vi "test Loopback with Disable.vi"(8 "error in":errorcluster, 11 "TestCase in":refnum<class "SingleCore.lvclass">) -> (0 "error out":errorcluster, 3 "TestCase out":refnum<class "SingleCore.lvclass">)   [LabVIEW 2020, in "SingleCore.lvclass"]
uses:
  SingleCore.lvclass
  C:/Git/niveristand-custom-device-testing-tools/VeriStandTestCase/VeriStandTestCase.lvclass
  4b06c685-66bb-4135-9ad1-d89a50a95502.vi
  <vilib>/numeric/Random Number (Range) I64.vi
  4cc353ea-8eb2-4b69-8f0e-bf7f0ec9a5d6.vi
  2771a990-9a12-45e1-bfa9-cf8078c77ee0.vi
  97c2081a-a4c0-4f2f-8a1c-7834fbf3da42.vi
  194ce8b8-c6d7-4123-a4fb-3c321acd640d.vi
  f114cf08-2618-4622-be37-923f8c3475b2.vi
  639b215b-9681-4d6c-ae13-b880b31cf4b5.vi
  f8fda0d9-e382-4aa3-871a-597408bfcf2f.vi
  <vilib>/numeric/sub_Random U32.vi
  <vilib>/NI VeriStand/Execution/Workspace/NI VeriStand - Set Multiple Channel Values.vi
  <vilib>/NI VeriStand/Execution/Workspace/NI VeriStand - Get Multiple Channel Values.vi
  <vilib>/addons/_JKI Toolkits/VI Tester/TestCase.llb/TestCase.lvclass
  <vilib>/NI VeriStand/Execution/Workspace/NI_VS Workspace ExecutionAPI.lvlib
  C:/Program Files (x86)/National Instruments/LabVIEW 2020/vi.lib/addons/_JKI Toolkits/VI Tester/TestCase.llb/TestCase.lvclass
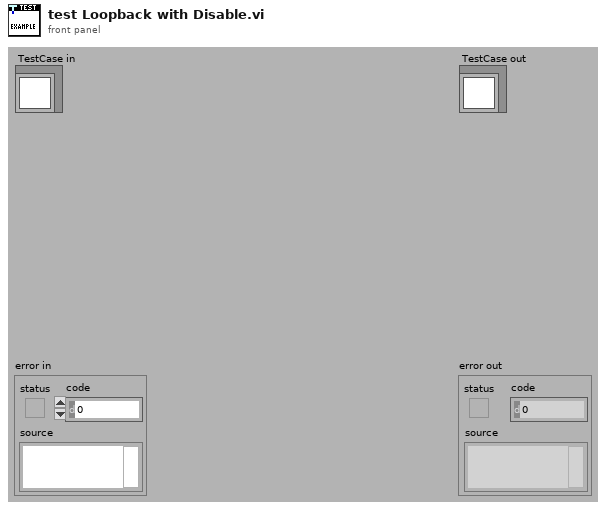
[diagram p1: front panel]
types:
  T1 = typedef "NI_VS Workspace ExecutionAPI.lvlib/WorkspaceAPI.ctl" = refnum<k24>
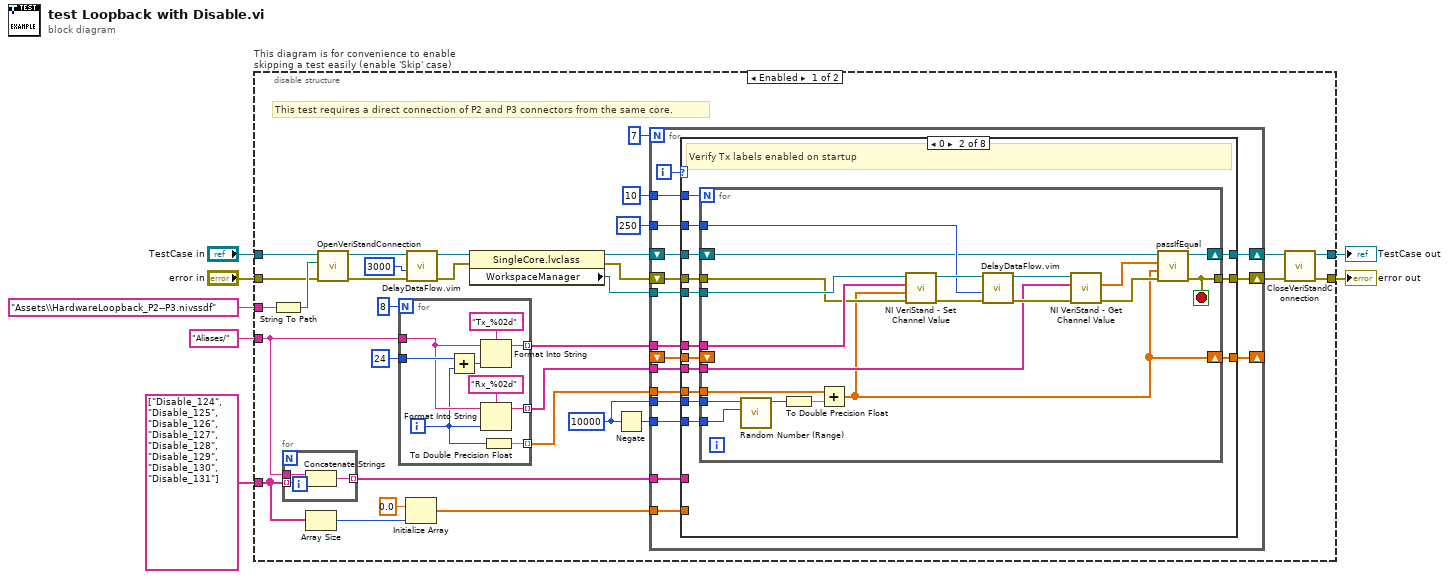
[diagram p0: block diagram]
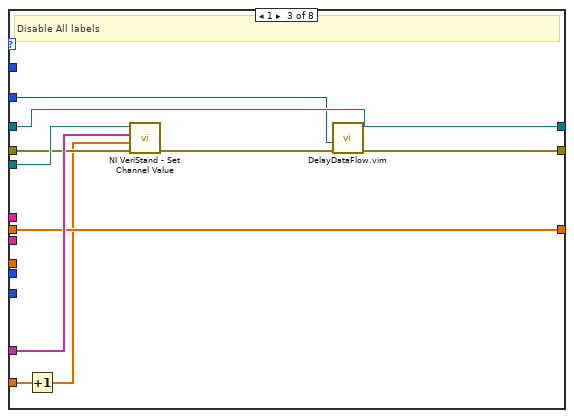
[diagram p3: hidden frame]
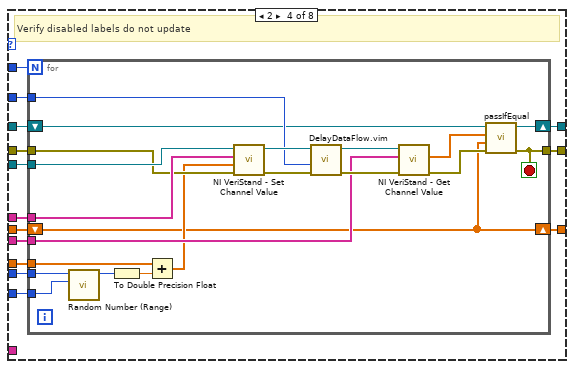
[diagram p4: hidden frame]
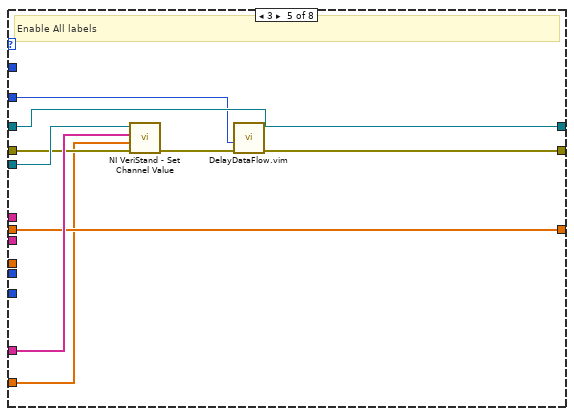
[diagram p5: hidden frame]
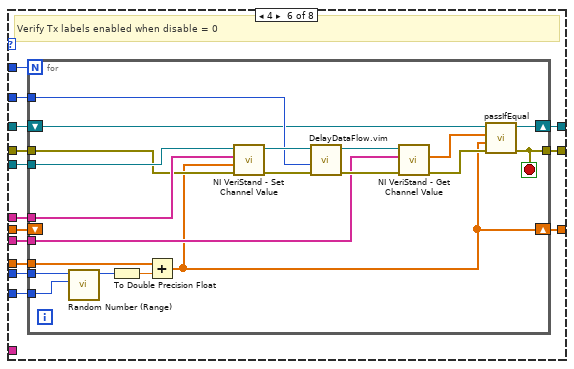
[diagram p6: hidden frame]
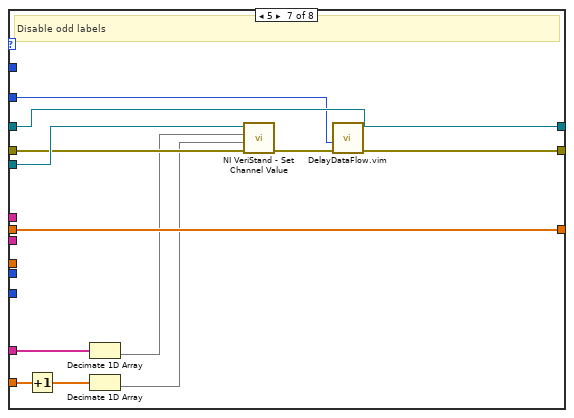
[diagram p7: hidden frame]
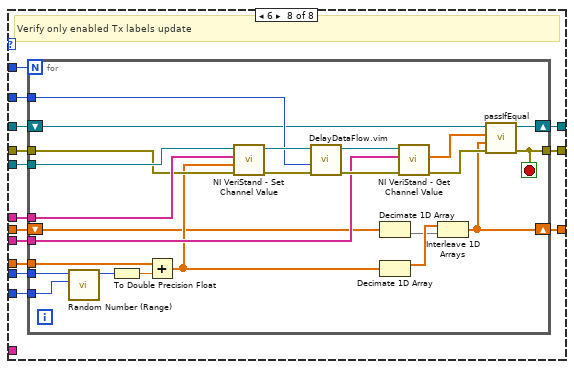
[diagram p8: hidden frame]
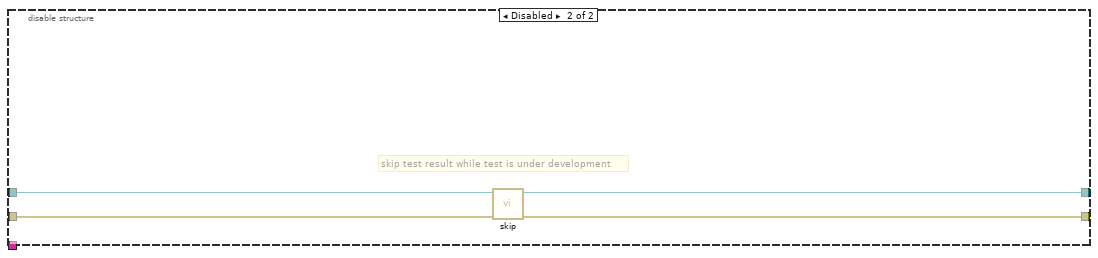
[diagram p9: hidden frame]
diagram:
  n1 = disable-structure "This diagram is for convenience to enable skipping a test easily (enable 'Skip' case)" shown="Enabled" {
    disable-tunnel: "TestCase in" -> [w33 w242]
    disable-tunnel: [w30 w240] -> w4
    disable-tunnel: [w29 w241] -> w6
    disable-tunnel: "error in" -> [w32 w239]
    disable-tunnel: "Assets\\HardwareLoopback_P2--P3.nivssdf" ("Channel") -> [w31 _]
    disable-tunnel: string[] ["Disable_124", "Disable_125", "Disable_126", "Disable_127", "Disable_128", "Disable_129", "Disable_130", "Disable_131"] -> [w13 _]
    disable-tunnel: "Aliases/" ("Channel") -> [w8 _]
    frame Enabled {
      w25 = i64 10000 ("upper bound (100)")
      # "This test requires a direct connection of P2 and P3 connectors from the same core."
      n2 = String To Path(string=w31) -> (path=w34:path)
      n3 = for {
        tunnel: w8 -> [w41]
        tunnel: w13 -> [w40] mode=indexing
        tunnel: [w39] -> w14 mode=indexing
        n4 = Concatenate Strings(w41, w40) -> (w39:string)
      }
      n5 = Array Size(array=w13) -> (size(s)=w12:i32)
      n6 = call-dynamic "OpenVeriStandConnection.vi"("error in (no error)"=w32, "System Definition File"=w34, "VeriStand Test Case in"=w33) -> ("error out"=w36:errorcluster, "VeriStand Test Case out"=w38:refnum<class "SingleCore.lvclass">)  [unwired: 6 in, 1 out]
      n7 = for {
        N: 8 -> [_]
        tunnel: 24 ("x") -> [w238]
        tunnel: w8 -> [w234]
        tunnel: [w233] -> w23 mode=indexing
        tunnel: [w231] -> w18 mode=indexing
        tunnel: [w230] -> w26 mode=indexing
        i -> [w232]
        n8 = Add(x=w238, y=w232) -> (x+y=w235:i32)
        n9 = Format Into String(format string="Tx_%02d", initial string=w234, w235) -> (resulting string=w233:string)  [unwired: 1 in, 1 out]
        n10 = Format Into String(format string="Rx_%02d", initial string=w234, w232) -> (resulting string=w231:string)  [unwired: 1 in, 1 out]
        n11 = To Double Precision Float(number=w232) -> (double precision float=w230:dbl)
      }
      n12 = Initialize Array(0.0 ("element"), w12) -> (w10:dbl[])
      n13 = call "DelayDataFlow.vim"("value in"=w36, "milliseconds to wait"=u32 3000) -> ("value out"=w35:errorcluster)  [unwired: 2 in, 1 out]
      n14 = property class="SingleCore.lvclass"(reference=w38, error in=w35) -> (reference out=w17:refnum<class "SingleCore.lvclass">, error out=w19:errorcluster, "WorkspaceManager"=w22:T1)
      n15 = Negate(x=w25) -> (-x=w24:i64)
      n16 = for {
        N: 7 -> [_]
        tunnel: w26 -> [w58]
        tunnel: w25 -> [w57]
        tunnel: w24 -> [w56]
        tunnel: w23 -> [w55]
        tunnel: w22 -> [w54]
        tunnel: 10 -> [w53]
        tunnel: u32 250 ("milliseconds to wait") -> [w52]
        tunnel: w18 -> [w50]
        shift-right: [w47] -> w15
        shift-left: w19 -> [w51]
        shift-right: [w48] -> w16
        shift-left: w17 -> [w49]
        tunnel: w14 -> [w45]
        tunnel: w10 -> [w44]
        shift-right: [w43] -> _
        shift-left: _ -> [w42]
        i -> [w46]
        n17 = case shown="0" w46 {
          tunnel: w58 -> [_ w75 _ w118 _ w161 _ w206]
          tunnel: w57 -> [_ w74 _ w117 _ w160 _ w205]
          tunnel: w56 -> [_ w73 _ w116 _ w159 _ w204]
          tunnel: w55 -> [_ w72 _ w115 _ w158 _ w203]
          tunnel: w54 -> [_ w71 w104 w114 w147 w157 w192 w202]
          tunnel: w53 -> [_ w70 _ w113 _ w156 _ w201]
          tunnel: w52 -> [_ w69 w98 w112 w141 w155 w187 w200]
          tunnel: w51 -> [w60 w68 w102 w111 w145 w154 w191 w199]
          tunnel: w50 -> [_ w67 _ w110 _ w153 _ w198]
          tunnel: w49 -> [w61 w66 w100 w109 w144 w152 w189 w197]
          tunnel: [w61 w65 w100 w108 w144 w151 w189 w196] -> w48
          tunnel: [w60 w64 w99 w107 w142 w150 w188 w195] -> w47
          tunnel: w45 -> [_ _ w103 _ w146 _ w182 _]
          tunnel: w44 -> [_ _ w101 _ w139 _ w190 _]
          tunnel: [w59 w63 w97 w105 w140 w149 w186 w194] -> w43
          tunnel: w42 -> [w59 w62 w97 w106 w140 w148 w186 w193]
          frame Default {
          }
          frame 0 {
            # "Verify Tx labels enabled on startup"
            n18 = for {
              N: w70 -> [_]
              tunnel: w75 -> [w89]
              tunnel: w74 -> [w88]
              tunnel: w73 -> [w87]
              tunnel: w72 -> [w86]
              tunnel: w71 -> [w85]
              tunnel: w69 -> [w84]
              tunnel: w68 -> [w83]
              tunnel: w67 -> [w82]
              shift-right: [w79] -> w65
              shift-left: w66 -> [w80]
              tunnel: [w77] -> w64
              shift-right: [w76] -> w63
              shift-left: w62 -> [_]
              stop <- w77 stop-if-true
              n19 = call-poly <vilib>:"Random Number (Range).vi"("lower bound (-100)"=w87, "upper bound (100)"=w88) -> ("number"=w91:i64)  [unwired: 9 in]
              n20 = To Double Precision Float(number=w91) -> (double precision float=w90:dbl)
              n21 = Add(x=w89, y=w90) -> (x+y=w76:dbl[])
              n22 = call-poly <vilib>:"NI VeriStand - Set Channel Value.vi"("error in (no error)"=w83, "Values"=w76, "Channels"=w86, "WorkspaceManager in"=w85) -> ("error out"=w93:errorcluster, "WorkspaceManager out"=w92:T1)  [unwired: 6 in]
              n23 = call "DelayDataFlow.vim"("value in"=w93, "milliseconds to wait"=w84) -> ("value out"=w94:errorcluster)  [unwired: 2 in, 1 out]
              n24 = call-poly <vilib>:"NI VeriStand - Get Channel Value.vi"("error in (no error)"=w94, "Channels"=w82, "WorkspaceManager in"=w92) -> ("error out"=w81:errorcluster, "Values"=w78:dbl[])  [unwired: 6 in, 1 out]
              n25 = call-dynamic "passIfEqual.vi"("error in (no error)"=w81, "y"=w76, "x"=w78, "TestCase in"=w80) -> ("error out"=w77:errorcluster, "TestCase out"=w79:refnum<class "SingleCore.lvclass">)  [unwired: 6 in]
            }
          }
          frame 1 {
            # "Disable All labels"
            n26 = Increment(x=w101) -> (x+1=w96:dbl[])
            n27 = call-poly <vilib>:"NI VeriStand - Set Channel Value.vi"("error in (no error)"=w102, "Values"=w96, "Channels"=w103, "WorkspaceManager in"=w104) -> ("error out"=w95:errorcluster)  [unwired: 6 in, 1 out]
            n28 = call "DelayDataFlow.vim"("value in"=w95, "milliseconds to wait"=w98) -> ("value out"=w99:errorcluster)  [unwired: 2 in, 1 out]
          }
          frame 2 {
            # "Verify disabled labels do not update"
            n29 = for {
              N: w113 -> [_]
              tunnel: w118 -> [w133]
              tunnel: w117 -> [w132]
              tunnel: w116 -> [w131]
              tunnel: w115 -> [w130]
              tunnel: w114 -> [w129]
              tunnel: w112 -> [w128]
              tunnel: w111 -> [w127]
              tunnel: w110 -> [w126]
              shift-right: [w123] -> w108
              shift-left: w109 -> [w124]
              tunnel: [w120] -> w107
              shift-right: [w119] -> w105
              shift-left: w106 -> [w119]
              stop <- w120 stop-if-true
              n30 = call-poly <vilib>:"Random Number (Range).vi"("lower bound (-100)"=w131, "upper bound (100)"=w132) -> ("number"=w135:i64)  [unwired: 9 in]
              n31 = To Double Precision Float(number=w135) -> (double precision float=w134:dbl)
              n32 = Add(x=w133, y=w134) -> (x+y=w121:dbl[])
              n33 = call-poly <vilib>:"NI VeriStand - Set Channel Value.vi"("error in (no error)"=w127, "Values"=w121, "Channels"=w130, "WorkspaceManager in"=w129) -> ("error out"=w137:errorcluster, "WorkspaceManager out"=w136:T1)  [unwired: 6 in]
              n34 = call "DelayDataFlow.vim"("value in"=w137, "milliseconds to wait"=w128) -> ("value out"=w138:errorcluster)  [unwired: 2 in, 1 out]
              n35 = call-poly <vilib>:"NI VeriStand - Get Channel Value.vi"("error in (no error)"=w138, "Channels"=w126, "WorkspaceManager in"=w136) -> ("error out"=w125:errorcluster, "Values"=w122:dbl[])  [unwired: 6 in, 1 out]
              n36 = call-dynamic "passIfEqual.vi"("error in (no error)"=w125, "y"=w119, "x"=w122, "TestCase in"=w124) -> ("error out"=w120:errorcluster, "TestCase out"=w123:refnum<class "SingleCore.lvclass">)  [unwired: 6 in]
            }
          }
          frame 3 {
            # "Enable All labels"
            n37 = call-poly <vilib>:"NI VeriStand - Set Channel Value.vi"("error in (no error)"=w145, "Values"=w139, "Channels"=w146, "WorkspaceManager in"=w147) -> ("error out"=w143:errorcluster)  [unwired: 6 in, 1 out]
            n38 = call "DelayDataFlow.vim"("value in"=w143, "milliseconds to wait"=w141) -> ("value out"=w142:errorcluster)  [unwired: 2 in, 1 out]
          }
          frame 4 {
            # "Verify Tx labels enabled when disable = 0"
            n39 = for {
              N: w156 -> [_]
              tunnel: w161 -> [w175]
              tunnel: w160 -> [w174]
              tunnel: w159 -> [w173]
              tunnel: w158 -> [w172]
              tunnel: w157 -> [w171]
              tunnel: w155 -> [w170]
              tunnel: w154 -> [w169]
              tunnel: w153 -> [w168]
              shift-right: [w165] -> w151
              shift-left: w152 -> [w166]
              tunnel: [w163] -> w150
              shift-right: [w162] -> w149
              shift-left: w148 -> [_]
              stop <- w163 stop-if-true
              n40 = call-poly <vilib>:"Random Number (Range).vi"("lower bound (-100)"=w173, "upper bound (100)"=w174) -> ("number"=w177:i64)  [unwired: 9 in]
              n41 = To Double Precision Float(number=w177) -> (double precision float=w176:dbl)
              n42 = Add(x=w175, y=w176) -> (x+y=w162:dbl[])
              n43 = call-poly <vilib>:"NI VeriStand - Set Channel Value.vi"("error in (no error)"=w169, "Values"=w162, "Channels"=w172, "WorkspaceManager in"=w171) -> ("error out"=w179:errorcluster, "WorkspaceManager out"=w178:T1)  [unwired: 6 in]
              n44 = call "DelayDataFlow.vim"("value in"=w179, "milliseconds to wait"=w170) -> ("value out"=w180:errorcluster)  [unwired: 2 in, 1 out]
              n45 = call-poly <vilib>:"NI VeriStand - Get Channel Value.vi"("error in (no error)"=w180, "Channels"=w168, "WorkspaceManager in"=w178) -> ("error out"=w167:errorcluster, "Values"=w164:dbl[])  [unwired: 6 in, 1 out]
              n46 = call-dynamic "passIfEqual.vi"("error in (no error)"=w167, "y"=w162, "x"=w164, "TestCase in"=w166) -> ("error out"=w163:errorcluster, "TestCase out"=w165:refnum<class "SingleCore.lvclass">)  [unwired: 6 in]
            }
          }
          frame 5 {
            # "Disable odd labels"
            n47 = Increment(x=w190) -> (x+1=w183:dbl[])
            n48 = Decimate 1D Array(w182) -> (w184:string[])  [unwired: 1 out]
            n49 = Decimate 1D Array(w183) -> (w181:dbl[])  [unwired: 1 out]
            n50 = call-poly <vilib>:"NI VeriStand - Set Channel Value.vi"("error in (no error)"=w191, "Values"=w181, "Channels"=w184, "WorkspaceManager in"=w192) -> ("error out"=w185:errorcluster)  [unwired: 6 in, 1 out]
            n51 = call "DelayDataFlow.vim"("value in"=w185, "milliseconds to wait"=w187) -> ("value out"=w188:errorcluster)  [unwired: 2 in, 1 out]
          }
          frame 6 {
            # "Verify only enabled Tx labels update"
            n52 = for {
              N: w201 -> [_]
              tunnel: w206 -> [w224]
              tunnel: w205 -> [w223]
              tunnel: w204 -> [w222]
              tunnel: w203 -> [w221]
              tunnel: w202 -> [w220]
              tunnel: w200 -> [w219]
              tunnel: w199 -> [w218]
              tunnel: w198 -> [w217]
              shift-right: [w214] -> w196
              shift-left: w197 -> [w215]
              tunnel: [w212] -> w195
              shift-right: [w207] -> w194
              shift-left: w193 -> [w209]
              stop <- w212 stop-if-true
              n53 = call-poly <vilib>:"Random Number (Range).vi"("lower bound (-100)"=w222, "upper bound (100)"=w223) -> ("number"=w226:i64)  [unwired: 9 in]
              n54 = To Double Precision Float(number=w226) -> (double precision float=w225:dbl)
              n55 = Add(x=w224, y=w225) -> (x+y=w211:dbl[])
              n56 = call-poly <vilib>:"NI VeriStand - Set Channel Value.vi"("error in (no error)"=w218, "Values"=w211, "Channels"=w221, "WorkspaceManager in"=w220) -> ("error out"=w228:errorcluster, "WorkspaceManager out"=w227:T1)  [unwired: 6 in]
              n57 = call "DelayDataFlow.vim"("value in"=w228, "milliseconds to wait"=w219) -> ("value out"=w229:errorcluster)  [unwired: 2 in, 1 out]
              n58 = Decimate 1D Array(w209) -> (w208:dbl[])  [unwired: 1 out]
              n59 = Decimate 1D Array(w211) -> (w210:dbl[])  [unwired: 1 out]
              n60 = call-poly <vilib>:"NI VeriStand - Get Channel Value.vi"("error in (no error)"=w229, "Channels"=w217, "WorkspaceManager in"=w227) -> ("error out"=w216:errorcluster, "Values"=w213:dbl[])  [unwired: 6 in, 1 out]
              n61 = Interleave 1D Arrays(w210, w208) -> (w207:dbl[])
              n62 = call-dynamic "passIfEqual.vi"("error in (no error)"=w216, "y"=w207, "x"=w213, "TestCase in"=w215) -> ("error out"=w212:errorcluster, "TestCase out"=w214:refnum<class "SingleCore.lvclass">)  [unwired: 6 in]
            }
          }
        }
      }
      n63 = call-dynamic "CloseVeriStandConnection.vi"("error in (no error)"=w15, "VeriStand Test Case in"=w16) -> ("error out"=w29:errorcluster, "VeriStand Test Case out"=w30:refnum<class "SingleCore.lvclass">)  [unwired: 8 in]
    }
    frame Disabled {
      # "skip test result while test is under development"
      n64 = call <vilib>:"skip.vi"("error in (no error)"=w239, "TestCase in"=w242) -> ("error out"=w241:errorcluster, "TestCase out"=w240:refnum<class "SingleCore.lvclass">)  [unwired: 8 in]
    }
  }
  "error out" <- w6
  "TestCase out" <- w4
